vi "HW_Set_IO_Dir_on_ECU.vi"(2 "Error In":errorcluster, 3 "IO ports config":bool[](array[boolean])=[FALSE, FALSE, TRUE, TRUE], 4 "VISA resource name":refnum<visa-resource-name>="Tracker", 5 "IO inversion config.":u16) -> (0 "error out":errorcluster, 1 "VISA resource name out":refnum<visa-resource-name>="Tracker")   [LabVIEW 2016]
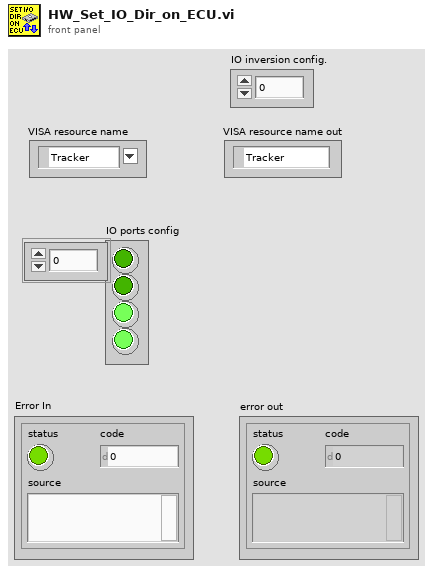
[diagram p1: front panel]
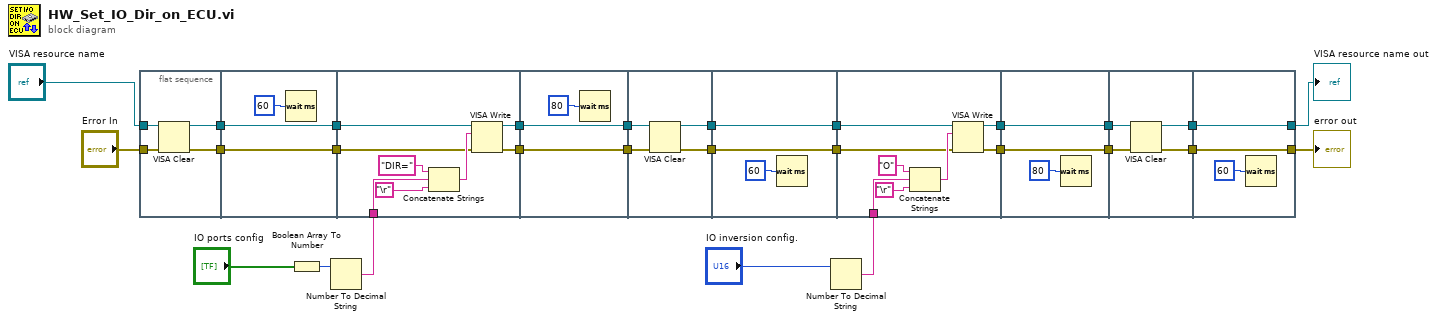
[diagram p0: block diagram]
diagram:
  n1 = flat-sequence {
    tunnel: "VISA resource name" -> [w31]
    tunnel: "Error In" -> [w30]
    tunnel: [w29] -> w23
    tunnel: [w28] -> w22
    tunnel: w23 -> [w33]
    tunnel: [w33] -> w21
    tunnel: [w32] -> w20
    tunnel: w22 -> [w32]
    tunnel: w21 -> [w40]
    tunnel: w20 -> [w39]
    tunnel: [w38] -> w19
    tunnel: [w37] -> w18
    tunnel: w15 -> [w35]
    tunnel: [w44] -> w17
    tunnel: w19 -> [w44]
    tunnel: [w43] -> w16
    tunnel: w18 -> [w43]
    tunnel: w17 -> [w49]
    tunnel: w16 -> [w48]
    tunnel: [w47] -> w14
    tunnel: [w46] -> w13
    tunnel: w14 -> [w52]
    tunnel: w13 -> [w51]
    tunnel: [w52] -> w12
    tunnel: [w51] -> w11
    tunnel: w12 -> [w57]
    tunnel: w11 -> [w56]
    tunnel: w9 -> [w55]
    tunnel: [w54] -> w7
    tunnel: [w53] -> w5
    tunnel: [w62] -> w8
    tunnel: w7 -> [w62]
    tunnel: [w61] -> w6
    tunnel: w5 -> [w61]
    tunnel: w8 -> [w67]
    tunnel: w6 -> [w66]
    tunnel: [w65] -> w3
    tunnel: [w64] -> w1
    tunnel: [w69] -> w4
    tunnel: w3 -> [w69]
    tunnel: [w68] -> w2
    tunnel: w1 -> [w68]
    frame #0 {
      n2 = VISA Clear(VISA resource name=w31, error in (no error)=w30) -> (VISA resource name out=w29:refnum<visa-resource-name>, error out=w28:errorcluster)
    }
    frame #1 {
      n3 = Wait (ms)(milliseconds to wait=u32 60) -> ()  [unwired: 1 out]
    }
    frame #2 {
      n4 = Concatenate Strings("DIR=" ("write buffer"), w35, "\r") -> (w42:string)
      n5 = VISA Write(VISA resource name=w40, write buffer=w42, error in (no error)=w39) -> (VISA resource name out=w38:refnum<visa-resource-name>, error out=w37:errorcluster)  [unwired: 1 out]
    }
    frame #3 {
      n6 = Wait (ms)(milliseconds to wait=u32 80) -> ()  [unwired: 1 out]
    }
    frame #4 {
      n7 = VISA Clear(VISA resource name=w49, error in (no error)=w48) -> (VISA resource name out=w46:refnum<visa-resource-name>, error out=w47:errorcluster)
    }
    frame #5 {
      n8 = Wait (ms)(milliseconds to wait=u32 60) -> ()  [unwired: 1 out]
    }
    frame #6 {
      n9 = Concatenate Strings("O" ("write buffer"), w55, "\r") -> (w60:string)
      n10 = VISA Write(VISA resource name=w56, write buffer=w60, error in (no error)=w57) -> (VISA resource name out=w54:refnum<visa-resource-name>, error out=w53:errorcluster)  [unwired: 1 out]
    }
    frame #7 {
      n11 = Wait (ms)(milliseconds to wait=u32 80) -> ()  [unwired: 1 out]
    }
    frame #8 {
      n12 = VISA Clear(VISA resource name=w67, error in (no error)=w66) -> (VISA resource name out=w65:refnum<visa-resource-name>, error out=w64:errorcluster)
    }
    frame #9 {
      n13 = Wait (ms)(milliseconds to wait=u32 60) -> ()  [unwired: 1 out]
    }
  }
  n14 = Boolean Array To Number(Boolean array="IO ports config") -> (number=w24:u32)
  n15 = Number To Decimal String(number=w24) -> (decimal integer string=w15:string)  [unwired: 1 in]
  n16 = Number To Decimal String(number="IO inversion config.") -> (decimal integer string=w9:string)  [unwired: 1 in]
  "error out" <- w2
  "VISA resource name out" <- w4
